vi "Write _regionSet.vi"(8 "error in (no error)":errorcluster, 10 "_regionSet?":bool, 11 "HTTP Request in":refnum<class "HTTP Request.lvclass">) -> (0 "error out":errorcluster, 3 "HTTP Request out":refnum<class "HTTP Request.lvclass">)   [LabVIEW 2015, in "NI_AWS_Core.lvlib" / "HTTP Request.lvclass"]
uses:
  HTTP Request.lvclass
  HTTP Request.lvclass/HTTP Request.ctl
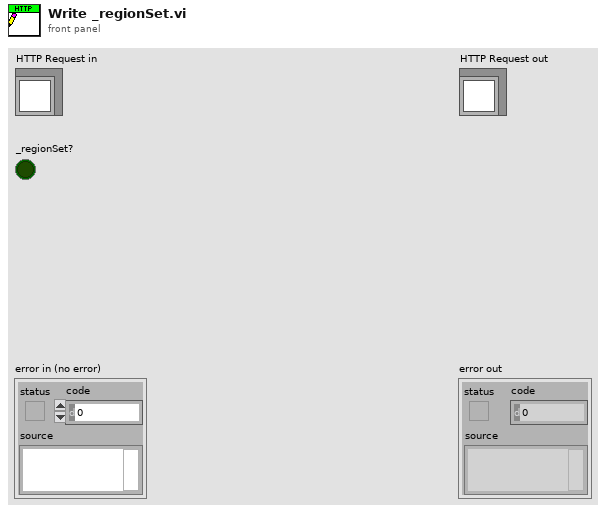
[diagram p1: front panel]
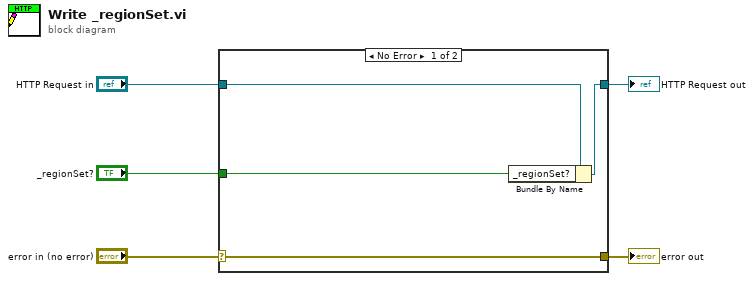
[diagram p0: block diagram]
diagram:
  n1 = case shown="No Error" "error in (no error)" {
    selector: "error in (no error)" -> [w9 w10]
    tunnel: [w9 w10] -> w4
    tunnel: [w7 w11] -> w2
    tunnel: "HTTP Request in" -> [w8 w11]
    tunnel: "_regionSet?" -> [w6 _]
    frame No Error {
      n2 = Bundle By Name(cluster=w8, "_regionSet?"=w6) -> (w7:refnum<class "HTTP Request.lvclass">)
    }
    frame Error {
    }
  }
  "error out" <- w4
  "HTTP Request out" <- w2
